vi "Define Target.vi"(8 "error in (no error)":errorcluster, 9 "Target Actor index(-1, all)":i32=-1, 10 "Target Actor":refnum<class "Actor.lvclass">, 11 "Targetted Msg in":refnum<class "Targetted Msg.lvclass">) -> (0 "error out":errorcluster, 3 "Targetted Msg out":refnum<class "Targetted Msg.lvclass">)   [LabVIEW 2020, in "Publisher.lvlib" / "Targetted Msg.lvclass"]
doc: "Configure 'Targetted Msg' for execution."
uses:
  Targetted Msg.lvclass
  PPL/HDH.Actor Framework.Core.Actor.lvlibp/1abvi3w/vi.lib/ActorFramework/Actor/Actor.lvclass
  Targetted Msg.lvclass/Targetted Msg.ctl
  PPL/HDH.Actor Framework.Core.Utility.lvlibp
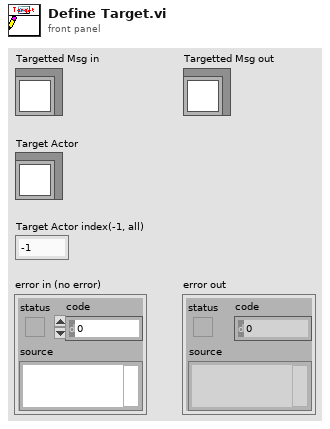
[diagram p1: front panel]
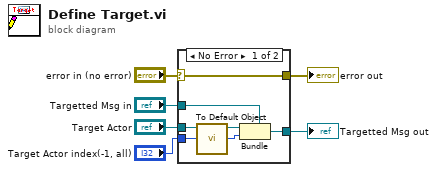
[diagram p0: block diagram]
diagram:
  n1 = case shown="No Error" "error in (no error)" {
    selector: "error in (no error)" -> [w7 w13]
    tunnel: [w7 w13] -> w5
    tunnel: [w12 w14] -> w3
    tunnel: "Targetted Msg in" -> [w8 w14]
    tunnel: "Target Actor" -> [w10 _]
    tunnel: "Target Actor index(-1, all)" -> [w11 _]
    frame No Error {
      n2 = call "To Default Object.vi"("Object in"=w10) -> ("Default out"=w9:refnum<class "Actor.lvclass">)  [unwired: 10 in]
      n3 = Bundle(cluster=w8, w9, w11) -> (w12:refnum<class "Targetted Msg.lvclass">)
    }
    frame Error {
    }
  }
  "error out" <- w5
  "Targetted Msg out" <- w3
